vi "Util.Pic.GIF.Write.Pack.Data.NormalizeImage.vi"(9 "bottom":i16, 10 "right":i16, 11 "image in":u8[](array[numeric])) -> (3 "image out":u8[](array[numeric]))   [LabVIEW 2014]
panel:
  # "Util.Pic.GIF.Write.Pack.Data.NormalizeImage.vi\n\nDetects and removes row-padding bytes.\n\nPlease visit http://www.OpenG.org to learn about the\nOpen Source LabVIEW software movement.\n\nNOTICE -- YOU MUST LEAVE THIS NOTICE IN PLACE.  PER THE TERMS OF THE LICENSE BELOW, YOU MAY SUBLICENSE THIS SOFTWARE \nIN ANY WAY THAT DOES NOT CONFLICT WITH THIS LICENSE.\n\n### BSD License (http://www.opensource.org/licenses/bsd-license.php) Begin ###\n \nCopyright (c) 2007, Bill Clench <bclench@yahoo.com>\n\nAll rights reserved.\n\nRedistribution and use in source and binary forms, with or without modification, are permitted provided that the following conditions are met:\n\n    * Redistributions of source code must retain the above copyright notice, this list of conditions and the following disclaimer.\n    * Redistributions in binary form must reproduce the above copyright notice, this list of conditions and the following disclaimer in the \n       documentation and/or other materials provided with the distribution.\n\nTHIS SOFTWARE IS PROVIDED BY THE COPYRIGHT HOLDERS AND CONTRIBUTORS \"AS IS\" AND ANY EXPRESS OR IMPLIED WARRANTIES, \nINCLUDING, BUT NOT LIMITED TO, THE IMPLIED WARRANTIES OF MERCHANTABILITY AND FITNESS FOR A PARTICULAR PURPOSE ARE \nDISCLAIMED. IN NO EVENT SHALL THE COPYRIGHT OWNER OR CONTRIBUTORS BE LIABLE FOR ANY DIRECT, INDIRECT, INCIDENTAL,\n SPECIAL, EXEMPLARY, OR CONSEQUENTIAL DAMAGES (INCLUDING, BUT NOT LIMITED TO, PROCUREMENT OF SUBSTITUTE GOODS OR \nSERVICES; LOSS OF USE, DATA, OR PROFITS; OR BUSINESS INTERRUPTION) HOWEVER CAUSED AND ON ANY THEORY OF LIABILITY, \nWHETHER IN CONTRACT, STRICT LIABILITY, OR TORT (INCLUDING NEGLIGENCE OR OTHERWISE) ARISING IN ANY WAY OUT OF THE USE \nOF THIS SOFTWARE, EVEN IF ADVISED OF THE POSSIBILITY OF SUCH DAMAGE.\n\n### BSD License End ###"
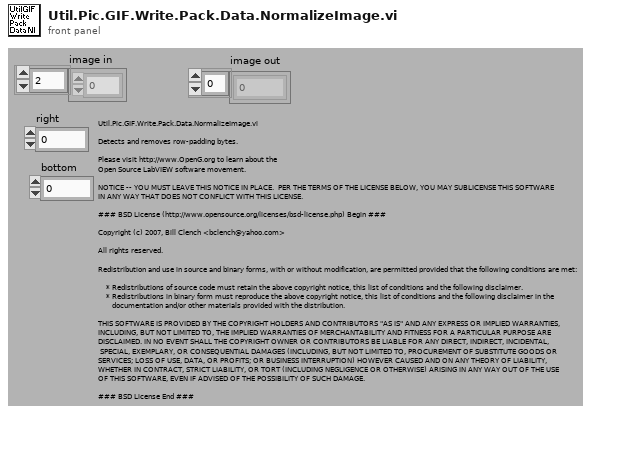
[diagram p1: front panel]
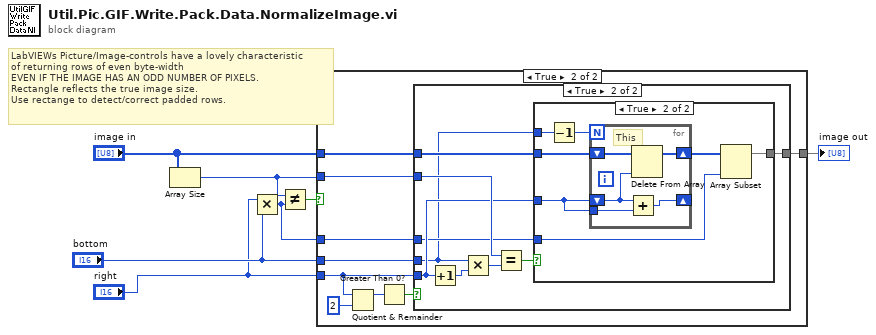
[diagram p0: block diagram]
diagram:
  # "LabVIEWs Picture/Image-controls have a lovely characteristic\nof returning rows of even byte-width\nEVEN IF THE IMAGE HAS AN ODD NUMBER OF PIXELS.\nRectangle reflects the true image size.\nUse rectange to detect/correct padded rows."
  n1 = Array Size(array="image in") -> (size(s)=w6:i32)
  n2 = Multiply(x="right", y="bottom") -> (x*y=w3:i16)
  n3 = Not Equal?(x=w6, y=w3) -> (x != y?=w7:bool)
  n4 = case shown="True" w7 {
    tunnel: "right" -> [_ w14]
    tunnel: "bottom" -> [_ w13]
    tunnel: w6 -> [_ w12]
    tunnel: "image in" -> [w8 w11]
    tunnel: [w8 w10] -> w4
    tunnel: w3 -> [_ w9]
    frame False {
    }
    frame True {
      n5 = Quotient & Remainder(x=w14, y=i16 2) -> (x-y*floor(x/y)=w16:i16)  [unwired: 1 out]
      n6 = Greater Than 0?(x=w16) -> (x > 0?=w15:bool)
      n7 = case shown="True" w15 {
        tunnel: w14 -> [_ w21]
        tunnel: w13 -> [_ w19]
        tunnel: w12 -> [_ w26]
        tunnel: w11 -> [w18 w25]
        tunnel: [w18 w23] -> w10
        tunnel: w9 -> [_ w20]
        frame False {
        }
        frame True {
          n8 = Increment(x=w21) -> (x+1=w22:i16)
          n9 = Multiply(x=w19, y=w22) -> (x*y=w27:i16)
          n10 = Equal?(x=w26, y=w27) -> (x = y?=w24:bool)
          n11 = case shown="True" w24 {
            tunnel: w25 -> [w28 w35]
            tunnel: [w28 w32] -> w23
            tunnel: w21 -> [_ w31]
            tunnel: w20 -> [_ w33]
            tunnel: w19 -> [_ w29]
            frame False {
            }
            frame True {
              n12 = Decrement(x=w29) -> (x-1=w30:i16)
              n13 = for {
                N: w30 -> [_]
                shift-right: [w36] -> w34
                shift-left: w35 -> [w40]
                shift-right: [w37] -> _
                shift-left: w31 -> [w39]
                tunnel: w31 -> [w38]
                # "This"
                n14 = Add(x=w39, y=w38) -> (x+y=w37:i16)
                n15 = Delete From Array(array=w40, index=w39) -> (array with subset deleted=w36:u8[])  [unwired: 1 in, 1 out]
              }
              n16 = Array Subset(array=w34, length=w33) -> (w32:u8[])  [unwired: 1 in]
            }
          }
        }
      }
    }
  }
  "image out" <- w4
